vi "Indexer.vi"(9 "Boolean 2":bool, 10 "Boolean":bool, 11 "refnum name":string) -> ()   [LabVIEW 2014]
uses:
  <vilib>/Rock Robotics/WPI/Relay/WPI_RelayValue.ctl
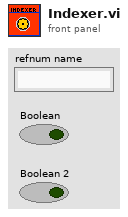
[diagram p1: front panel]
types:
  T1 = typedef "WPI_RelayValue.ctl" = enum16{"Off", "On", "Forward", "Reverse"}
  T2 = typedef "WPI_RelayDevRef.ctl" = cluster{"DevStatus":errorcluster, "Relay Channel":T3, "Controller":T4, "Relay Direction":T5}
  T3 = typedef "FPGA_DIORelayChannel.ctl" = enum8{"Relay 0", "Relay 1", "Relay 2", "Relay 3", "Invalid"}
  T4 = typedef "FPGA_TypedefDigitalModule.ctl" = enum16{"Controller 1"}
  T5 = typedef "WPI_RelayDirection.ctl" = enum16{"Both directions", "Forward only", "Reverse only"}
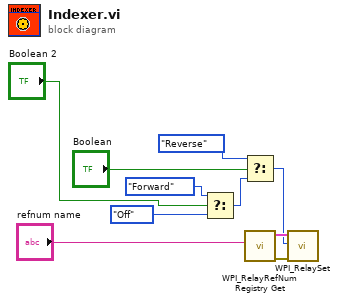
[diagram p0: block diagram]
diagram:
  n1 = Select(t=WPI_RelayValue."Forward" ("RelayValue"), s="Boolean 2", f=WPI_RelayValue."Off" ("RelayValue")) -> (s? t:f=w3:T1)
  n2 = Select(t=WPI_RelayValue."Reverse" ("RelayValue"), s="Boolean", f=w3) -> (s? t:f=w1:T1)
  n3 = call <vilib>:"WPI_RelayRefNum Registry Get.vi"("refnum name"="refnum name") -> ("error out"=w7:errorcluster, "RelayDevRef"=w8:T2)  [unwired: 9 in]
  n4 = call <vilib>:"WPI_RelaySet.vi"("error in (no error)"=w7, "RelayValue"=w1, "RelayDevRef"=w8) -> ()  [unwired: 7 in, 2 out]
